vi "Word Find Replace.vi"(8 "error in (no error)":errorcluster, 9 "Mathcad Output":T2, 10 "DesignRequest":T1, 11 "Word Doc":refnum<k7>) -> (0 "error out":errorcluster, 1 "Find-Replace":cluster{"Find":string, "Replace":string}[](array[cluster]), 2 "DesignRequest out":T1, 3 "Word Doc out":refnum<k7>)   [LabVIEW 2012, in "Design Server.lvlib"]
uses:
  Design Server.lvlib
  Design Request.ctl
  Variable cluster.ctl
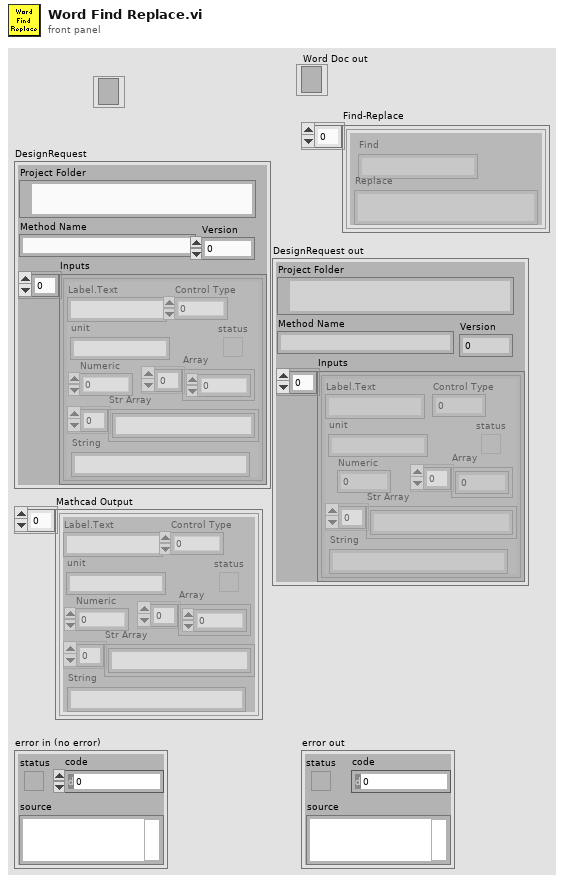
[diagram p1: front panel]
types:
  T1 = typedef "Design Server.lvlib/Design Request.ctl" = cluster{"Project Folder":path, "Method Name":string, "Inputs":T2, "Version":i32}
  T2 = typedef "Design Server.lvlib/Variable cluster.ctl" = cluster{"Label.Text":string, "Control Type":u32, "Numeric":dbl, "Array":dbl[], "status":bool, "Str Array":string[], "String":string, "unit":string}[]
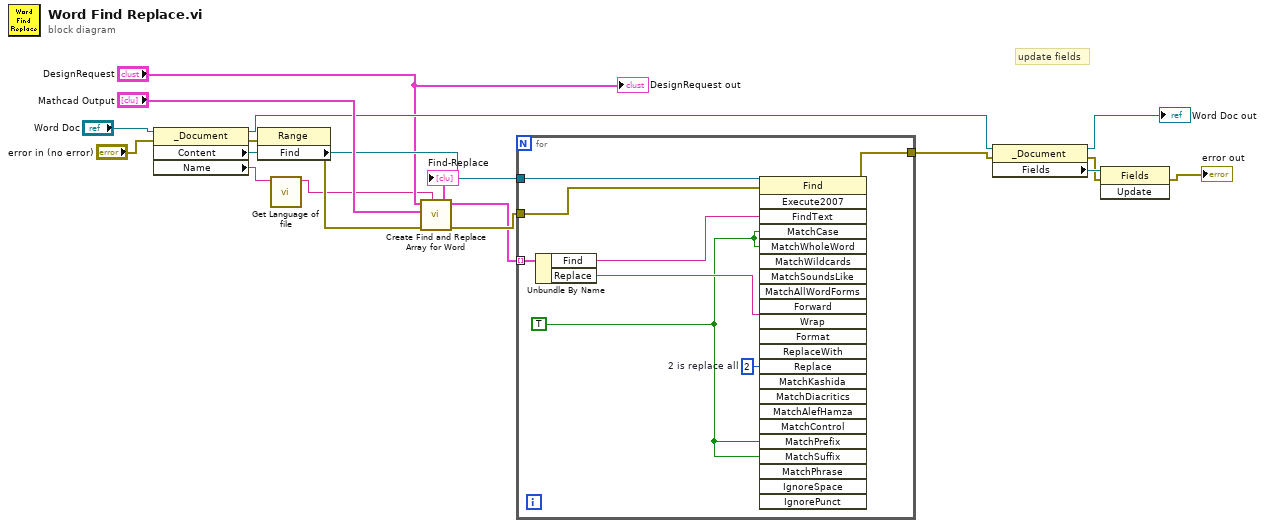
[diagram p0: block diagram]
diagram:
  # "update fields"
  n1 = property class="_Document"(reference="Word Doc", error in="error in (no error)") -> (reference out=w5:refnum<k7>, error out=w13:errorcluster, "Content"=w12:refnum<k7>, "Name"=w2:string)
  n2 = property class="Range"(reference=w12, error in=w13) -> (error out=w16:errorcluster, "Find"=w11:refnum<k7>)  [unwired: 1 out]
  n3 = call "Get Language of file.vi"("FileName"=w2) -> ("substring before match"=w1:string)  [unwired: 10 in]
  n4 = call "Create Find and Replace Array for Word.vi"("Language"=w1, "error in"=w16, "Mathcad Output"="Mathcad Output", "DesignRequest"="DesignRequest") -> ("error out"=w17:errorcluster, "Find-Replace"=w15:cluster{"Find":string, "Replace":string}[])  [unwired: 6 in]
  "Find-Replace" <- w15
  n5 = for {
    tunnel: w11 -> [w26]
    tunnel: w17 -> [w25]
    tunnel: [w23] -> w7
    tunnel: w15 -> [w22] mode=indexing
    w19 = TRUE ("Visible")
    w24 = 2  # 2 is replace all
    n6 = Unbundle By Name(w22) -> ("Find"=w21:string, "Replace"=w20:string)
    n7 = invoke class="Find" method="Execute2007"(reference=w26, error in=w25, "FindText"=w21, "MatchCase"=w19, "MatchWholeWord"=w19, "ReplaceWith"=w20, "Replace"=w24, "MatchPrefix"=w19, "MatchSuffix"=w19) -> (error out=w23:errorcluster)  [unwired: 14 in, 22 out]
  }
  n8 = property class="_Document"(reference=w5, error in=w7) -> (reference out=→"Word Doc out":refnum<k7>, error out=w8:errorcluster, "Fields"=w9:refnum<k7>)
  n9 = invoke class="Fields" method="Update"(reference=w9, error in=w8) -> (error out=→"error out":errorcluster)  [unwired: 1 in, 2 out]
  "DesignRequest out" <- "DesignRequest"
